vi "Handle Packet Validation Error.vi"(9 "Packet Validation Error":errorcluster, 10 "ControlPacket":refnum<class "ControlPacket.lvclass">, 11 "Session in":refnum<class "Session.lvclass">) -> (0 "error out":errorcluster, 3 "Session out":refnum<class "Session.lvclass">)   [LabVIEW 2013, in "MQTT Server.lvlib" / "Session.lvclass"]
uses:
  Session.lvclass
  Control Packets/ControlPacket/ControlPacket.lvclass
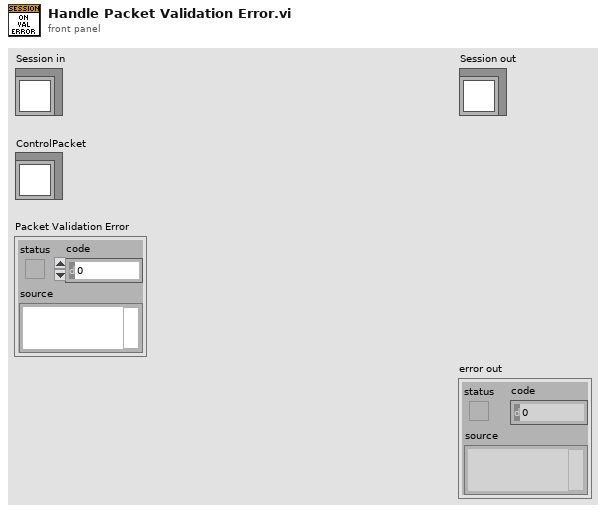
[diagram p1: front panel]
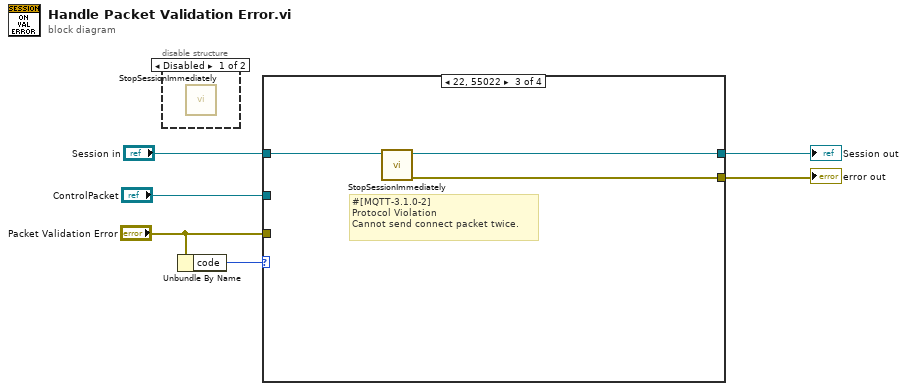
[diagram p0: block diagram]
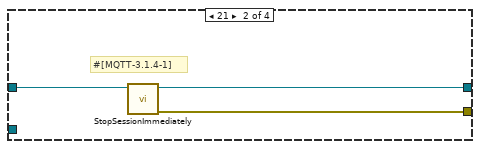
[diagram p4: hidden frame]
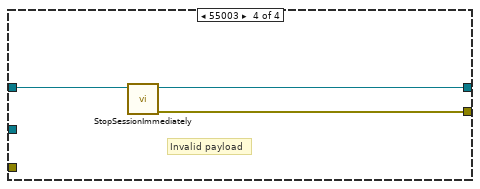
[diagram p5: hidden frame]
diagram:
  n1 = disable-structure shown="Disabled" {
    frame Disabled {
      n2 = call "StopSessionImmediately.vi"() -> ()  [unwired: 10 in, 2 out]
    }
    frame Enabled {
    }
  }
  n3 = Unbundle By Name("Packet Validation Error") -> ("code"=w4:i32)
  n4 = case shown="22, 55022" w4 {
    tunnel: "Session in" -> [w7 w10 w13 w16]
    tunnel: "ControlPacket" -> [_ _ _ _]
    tunnel: "Packet Validation Error" -> [_ _ _ _]
    tunnel: [w7 w9 w12 w15] -> w2
    tunnel: [_ w8 w11 w14] -> w1
    frame Default {
    }
    frame 21 {
      # "#[MQTT-3.1.4-1]"
      n5 = call "StopSessionImmediately.vi"("Session in"=w10) -> ("error out"=w8:errorcluster, "Session out"=w9:refnum<class "Session.lvclass">)  [unwired: 9 in]
    }
    frame 22, 55022 {
      # "#[MQTT-3.1.0-2]\nProtocol Violation\nCannot send connect packet twice."
      n6 = call "StopSessionImmediately.vi"("Session in"=w13) -> ("error out"=w11:errorcluster, "Session out"=w12:refnum<class "Session.lvclass">)  [unwired: 9 in]
    }
    frame 55003 {
      # "Invalid payload"
      n7 = call "StopSessionImmediately.vi"("Session in"=w16) -> ("error out"=w14:errorcluster, "Session out"=w15:refnum<class "Session.lvclass">)  [unwired: 9 in]
    }
  }
  "error out" <- w1
  "Session out" <- w2
